vi "2 Ch Digital Input.vi"(2 "2 Ch Digital In":cluster{"DI0":refnum<k21>, "DI1":refnum<k21>}={"DI0"="Chassis1/Mod4/DI0", "DI1"="Chassis1/Mod4/DI0"}) -> (7 "Packet":u64)   [LabVIEW 2009]
uses:
  <vilib>/eio/EIONode/EIONode.xnode
  <vilib>/rvi/eio/nirviEIOImplementation/nirviEIOImplementation.xnode
  <vilib>/rvi/eio/common/nirviEmuTemplateMethod_noerrors.vi
  <vilib>/rvi/eio/common/nirviEmuClasses.ctl
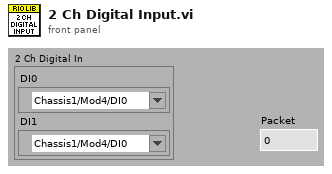
[diagram p1: front panel]
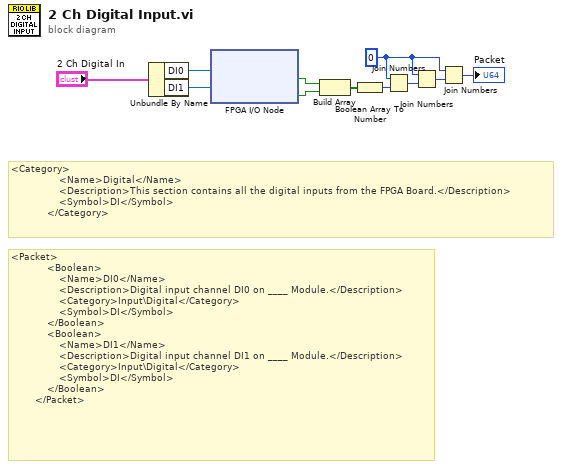
[diagram p0: block diagram]
diagram:
  w1 = u8 0 ("hi")
  # "<Category>\n                <Name>Digital</Name>\n                <Description>This section contains all the digital inputs from the FPGA Board.</Description>\n                <Symbol>DI</Symbol>\n            </Category>"
  # "<Packet>\n            <Boolean>\n                <Name>DI0</Name>\n                <Description>Digital input channel DI0 on ____ Module.</Description>\n                <Category>Input\\Digital</Category>\n                <Symbol>DI</Symbol>\n            </Boolean>\n            <Boolean>\n                <Name>DI1</Name>\n                <Description>Digital input channel DI1 on ____ Module.</Description>\n                <Category>Input\\Digital</Category>\n                <Symbol>DI</Symbol>\n            </Boolean>\n        </Packet>"
  n1 = Unbundle By Name("2 Ch Digital In") -> ("DI0"=w10:refnum<k21>, "DI1"=w11:refnum<k21>)
  n2 = xnode "FPGA I/O Node"("FPGA I/O In"=w10, "FPGA I/O In"=w11) -> ("I/O Item"=w7:bool, "I/O Item"=w8:bool)  [unwired: 2 out]
  n3 = Build Array(w7, w8) -> (w6:bool[])
  n4 = Boolean Array To Number(Boolean array=w6) -> (number=w5:u8)
  n5 = Join Numbers(hi=w1, lo=w5) -> ((hi.lo)=w4:u16)
  n6 = Join Numbers(hi=w1, lo=w4) -> ((hi.lo)=w3:u32)
  n7 = Join Numbers(hi=w1, lo=w3) -> ((hi.lo)=→"Packet":u64)
